vi "butterworth_lpf_tester.vi"() -> ()   [LabVIEW 2015]
uses:
  discrete_control_systems/discrete_control_systems.lvlib
  <vilib>/measure/NI_MABase.lvlib
  <vilib>/ptbypt/NI_PtbyPt.lvlib
panel:
  in  "Input Frequencies":T1(array[cluster])=[{"frequency"=10.0, "amplitude"=1.0, "phase"=0.0}, {"frequency"=100.0, "amplitude"=1.0, "phase"=0.0}, {"frequency"=250.0, "amplitude"=1.0, "phase"=0.0}]
  out "Frequency Chart":T2(graph)=[{[0.0, 1.0, 2.0, 3.0, 4.0, 5.0, 6.0, 7.0, 8.0, 9.0, 10.0, 11.0, 12.0, 13.0, 14.0, 15.0, 16.0, 17.0, 18.0, 19.0, 20.0, 21.0, 22.0, 23.0, 24.0, 25.0, 26.0, 27.0, 28.0, 29.0, 30.0, 31.0, 32.0, 33.0, 34.0, 35.0, 36.0, 37.0, 38.0, 39.0, 40.0, 41.0, 42.0, 43.0, 44.0, 45.0, 46.0, 47.0, 48.0, 49.0, 50.0, 51.0, 52.0, 53.0, 54.0, 55.0, 56.0, 57.0, 58.0, 59.0, 60.0, 61.0, 62.0, 63.0, 64.0, 65.0, 66.0, 67.0, 68.0, 69.0, 70.0, 71.0, 72.0, 73.0, 74.0, 75.0, 76.0, 77.0, 78.0, 79.0, 80.0, 81.0, 82.0, 83.0, 84.0, 85.0, 86.0, 87.0, 88.0, 89.0, 90.0, 91.0, 92.0, 93.0, 94.0, 95.0, 96.0, 97.0, 98.0, 99.0, 100.0, 101.0, 102.0, 103.0, 104.0, 105.0, 106.0, 107.0, 108.0, 109.0, 110.0, 111.0, 112.0, 113.0, 114.0, 115.0, 116.0, 117.0, 118.0, 119.0, 120.0, 121.0, 122.0, 123.0, 124.0, 125.0, 126.0, 127.0, 128.0, 129.0, 130.0, 131.0, 132.0, 133.0, 134.0, 135.0, 136.0, 137.0, 138.0, 139.0, 140.0, 141.0, 142.0, 143.0, 144.0, 145.0, 146.0, 147.0, 148.0, 149.0, 150.0, 151.0, 152.0, 153.0, 154.0, 155.0, 156.0, 157.0, 158.0, 159.0, 160.0, 161.0, 162.0, 163.0, 164.0, 165.0, 166.0, 167.0, 168.0, 169.0, 170.0, 171.0, 172.0, 173.0, 174.0, 175.0, 176.0, 177.0, 178.0, 179.0, 180.0, 181.0, 182.0, 183.0, 184.0, 185.0, 186.0, 187.0, 188.0, 189.0, 190.0, 191.0, 192.0, 193.0, 194.0, 195.0, 196.0, 197.0, 198.0, 199.0, 200.0, 201.0, 202.0, 203.0, 204.0, 205.0, 206.0, 207.0, 208.0, 209.0, 210.0, 211.0, 212.0, 213.0, 214.0, 215.0, 216.0, 217.0, 218.0, 219.0, 220.0, 221.0, 222.0, 223.0, 224.0, 225.0, 226.0, 227.0, 228.0, 229.0, 230.0, 231.0, 232.0, 233.0, 234.0, 235.0, 236.0, 237.0, 238.0, 239.0, 240.0, 241.0, 242.0, 243.0, 244.0, 245.0, 246.0, 247.0, 248.0, 249.0, 250.0, 251.0, 252.0, 253.0, 254.0, 255.0, 256.0, 257.0, 258.0, 259.0, 260.0, 261.0, 262.0, 263.0, 264.0, 265.0, 266.0, 267.0, 268.0, 269.0, 270.0, 271.0, 272.0, 273.0, 274.0, 275.0, 276.0, 277.0, 278.0, 279.0, 280.0, 281.0, 282.0, 283.0, 284.0, 285.0, 286.0, 287.0, 288.0, 289.0, 290.0, 291.0, 292.0, 293.0, 294.0, 295.0, 296.0, 297.0, 298.0, 299.0, 300.0, 301.0, 302.0, 303.0, 304.0, 305.0, 306.0, 307.0, 308.0, 309.0, 310.0, 311.0, 312.0, 313.0, 314.0, 315.0, 316.0, 317.0, 318.0, 319.0, 320.0, 321.0, 322.0, 323.0, 324.0, 325.0, 326.0, 327.0, 328.0, 329.0, 330.0, 331.0, 332.0, 333.0, 334.0, 335.0, 336.0, 337.0, 338.0, 339.0, 340.0, 341.0, 342.0, 343.0, 344.0, 345.0, 346.0, 347.0, 348.0, 349.0, 350.0, 351.0, 352.0, 353.0, 354.0, 355.0, 356.0, 357.0, 358.0, 359.0, 360.0, 361.0, 362.0, 363.0, 364.0, 365.0, 366.0, 367.0, 368.0, 369.0, 370.0, 371.0, 372.0, 373.0, 374.0, 375.0, 376.0, 377.0, 378.0, 379.0, 380.0, 381.0, 382.0, 383.0, 384.0, 385.0, 386.0, 387.0, 388.0, 389.0, 390.0, 391.0, 392.0, 393.0, 394.0, 395.0, 396.0, 397.0, 398.0, 399.0, 400.0, 401.0, 402.0, 403.0, 404.0, 405.0, 406.0, 407.0, 408.0, 409.0, 410.0, 411.0, 412.0, 413.0, 414.0, 415.0, 416.0, 417.0, 418.0, 419.0, 420.0, 421.0, 422.0, 423.0, 424.0, 425.0, 426.0, 427.0, 428.0, 429.0, 430.0, 431.0, 432.0, 433.0, 434.0, 435.0, 436.0, 437.0, 438.0, 439.0, 440.0, 441.0, 442.0, 443.0, 444.0, 445.0, 446.0, 447.0, 448.0, 449.0, 450.0, 451.0, 452.0, 453.0, 454.0, 455.0, 456.0, 457.0, 458.0, 459.0, 460.0, 461.0, 462.0, 463.0, 464.0, 465.0, 466.0, 467.0, 468.0, 469.0, 470.0, 471.0, 472.0, 473.0, 474.0, 475.0, 476.0, 477.0, 478.0, 479.0, 480.0, 481.0, 482.0, 483.0, 484.0, 485.0, 486.0, 487.0, 488.0, 489.0, 490.0, 491.0, 492.0, 493.0, 494.0, 495.0, 496.0, 497.0, 498.0, 499.0], "Power Spectrum (V^2 rms)"=[1.4416926080979755e-33, 7.826213800029281e-32, 3.9498488932288474e-32, 1.5451857789689928e-30, 1.770229960057915e-30, 1.69201989203789e-30, 2.7845850463504282e-30, 1.2307395944615857e-30, 3.884995553910035e-30, 5.168656132569903e-30, 0.4999999999999982, 1.969530656783117e-30, 1.1641495015956739e-32, 3.1610194499986036e-31, 3.906328330722268e-31, 1.457117797023426e-31, 1.330337649829857e-32, 6.461483253768492e-32, 1.5616698776899155e-32, 2.276840543231828e-32, 4.340384191049091e-32, 1.4612569748456343e-34, 2.009475244629669e-32, 1.6938033089417007e-32, 1.4069965949652836e-33, 2.9370893875103904e-34, 4.1778135170234854e-33, 5.139983465340829e-34, 3.565651291595972e-33, 1.1319414432831867e-33, 2.582687462864579e-33, 1.640047984930311e-33, 2.416435027087375e-33, 7.474025668657131e-34, 3.12677345736095e-33, 8.987590900801263e-33, 4.044144734420147e-34, 1.5808341132307828e-33, 1.5363072292167516e-32, 8.760300352472517e-34, 1.0177291753475116e-33, 5.3933988681594166e-33, 3.094430160245811e-33, 3.6514645669450685e-33, 1.845402037107353e-32, 5.966999353874168e-33, 8.386682269210854e-33, 7.536783251449749e-33, 2.7856650715616583e-33, 2.3536577227703477e-32, 6.94276482685008e-33, 7.125879164475322e-33, 4.4450660331730737e-32, 1.8424832517557833e-33, 3.2394696332391185e-32, 2.640596016281803e-32, 2.2137409152759435e-34, 2.984628117807155e-32, 3.715251366702514e-32, 8.523642080910707e-34, 3.518950726006882e-32, 3.0788156447005256e-32, 5.90445131225627e-33, 4.2742949035156564e-32, 4.4677630405293677e-32, 4.05918239542787e-33, 1.7399436600285105e-32, 3.7431449952700253e-32, 7.361354144680187e-33, 3.5112815188938977e-32, 7.714825459987569e-32, 9.56888278033162e-33, 6.891617057911108e-32, 2.901196216321453e-32, 9.942728893693235e-33, 6.820067373804319e-32, 7.66222569392888e-32, 9.778702524795351e-32, 7.459172896931001e-33, 2.6676613409008465e-32, 1.6078486549320684e-31, 4.553433334830302e-32, 5.967202732078624e-32, 1.6239147933409942e-31, 1.3496976214819333e-31, 3.9429831840891685e-32, 2.3879660230913693e-31, 5.368439062607186e-31, 5.768466483336905e-32, 1.2470806227799778e-32, 2.766251451204196e-31, 8.868922801342348e-31, 8.58630352129632e-31, 1.5210185871820127e-30, 1.3258487785965978e-30, 1.6197385144063318e-31, 1.2762558791513746e-30, 6.710012230270998e-30, 5.676225100951419e-30, 4.425084386122248e-29, 0.5000000000000158, 6.085550406083389e-29, 2.182023700085748e-29, 1.2206187767518531e-30, 2.0864465725220987e-30, 1.4770434620635963e-30, 3.523858426916773e-31, 7.93604350496358e-31, 2.565118914205842e-30, 1.7242628308667189e-31, 9.68545103065377e-31, 9.86323883154825e-32, 6.458420254775134e-31, 8.523139182093401e-32, 4.194413122625809e-31, 2.464847420841163e-31, 8.543898549846276e-32, 7.219309877932933e-32, 1.7906708675007333e-31, 4.6452074403981264e-32, 3.8477405557390846e-32, 3.035835051322331e-32, 1.2180170148794037e-31, 1.1146429562259039e-31, 6.476548031864476e-33, 8.650352863814154e-32, 4.792823037283406e-33, 7.436692826321392e-32, 1.2241937957673477e-32, 6.632121263130577e-32, 2.1380324550874632e-32, 4.143580651523067e-32, 8.799053144455967e-33, 1.0088347686413651e-32, 2.6983874731607125e-32, 6.628822838476204e-33, 2.6184364204135304e-32, 1.894787194962421e-32, 3.739693728815509e-33, 1.3373978008557082e-32, 6.624089673048897e-33, 4.0400771703784884e-33, 1.287914035386759e-33, 9.436354148245546e-33, 2.207627243261181e-33, 4.851741086145017e-34, 1.6218980211328037e-32, 6.589281185598417e-33, 1.7013683617642901e-32, 1.7443686766707493e-33, 5.763245210217634e-33, 5.65694620323976e-33, 8.631025771627826e-33, 2.5687283226277784e-33, 3.058043950990904e-33, 4.921629231963812e-33, 2.908234334710245e-33, 1.0920694549037408e-32, 3.462507728241332e-33, 1.107711087540309e-32, 5.609195466569585e-33, 6.162975822032968e-33, 6.76943729482967e-33, 6.812011131805112e-33, 5.5029211115021525e-33, 5.448070626678333e-33, 8.878235057809582e-33, 8.698966417095313e-33, 7.08882735383515e-33, 9.322166532213402e-33, 6.581787007004258e-33, 8.351078757892759e-33, 1.0268010757578787e-32, 1.1593617553095322e-32, 1.4267436939442722e-32, 6.226503776805651e-33, 9.345832359376988e-33, 1.1140811393499788e-32, 1.77715570804321e-32, 9.407881199960675e-33, 1.2642383474696908e-32, 2.2352990047032125e-32, 3.1882429782110666e-32, 4.0355165682688926e-33, 5.641464807976526e-33, 1.8364607917827892e-32, 3.5793700757787525e-32, 2.5934048778155828e-33, 1.283400271894388e-32, 3.2980721377406254e-32, 4.3911769725817854e-32, 4.6509513338604736e-33, 5.789672050545613e-33, 3.850282166966283e-32, 3.0009476777849937e-32, 9.266058800347179e-32, 3.6934714101451646e-33, 2.0164591288312445e-32, 5.897082858367753e-32, 9.435373618795044e-32, 5.983023091011311e-33, 2.8825575285456224e-32, 3.8039390539710766e-32, 1.4219318889417639e-31, 3.8445197845675e-33, 1.3808868397449647e-32, 9.7431723528794e-32, 1.2597261247197579e-31, 6.33494749937893e-33, 2.9949720564266167e-32, 7.733736551282448e-32, 1.5366164873435718e-31, 6.166451740396937e-33, 9.815204597979901e-33, 4.5732337435516326e-32, 1.6006431501198883e-31, 2.83957311411483e-31, 1.2373141549941634e-32, 7.202349368473215e-32, 2.0919361076481724e-31, 3.6135272599380592e-31, 6.013674651267553e-32, 7.876554887792541e-32, 2.1434495259467614e-31, 3.950611530668476e-31, 6.767304905202559e-32, 1.5526430748574623e-31, 2.849409038635409e-31, 5.417340072484559e-31, 3.542820085445006e-32, 1.6060656443977058e-31, 3.6131797297322066e-31, 7.814181997951294e-31, 6.70720664647277e-32, 1.1879744953070144e-31, 4.596993494460398e-31, 1.2844556938306713e-30, 2.4927911929223084e-30, 1.1357135696714613e-31, 6.407145162612521e-31, 2.1402927669151867e-30, 5.0308870470392406e-30, 2.170587773976856e-31, 1.4119777477564536e-30, 5.8193305652020806e-30, 1.7031719486667104e-29, 1.607219724884636e-30, 8.765652428972398e-30, 4.1926305807156045e-29, 3.6426071997166952e-28, 0.49999999999999956, 3.915928597894715e-29, 3.739525641719464e-29, 4.065046972439548e-29, 1.671275554714979e-30, 2.0701970633361013e-30, 4.356912241794652e-30, 6.308425787741234e-30, 8.575400552992506e-30, 3.016109187642351e-31, 1.0047009930537242e-30, 2.1368526862571695e-30, 3.281649862910867e-30, 8.007998836129683e-32, 4.7823844969883745e-31, 9.76487434778471e-31, 1.7079840097022587e-30, 1.72527962943393e-32, 1.9609726865406507e-31, 5.857500529853116e-31, 1.3969367464170784e-30, 2.2947224175787007e-33, 1.074143145500021e-31, 4.3685243386464885e-31, 7.196210120103431e-31, 1.952401774436985e-32, 7.186988767530748e-32, 1.2087302115028595e-31, 5.367618647260577e-31, 8.8410306518793e-31, 1.4671241278284904e-32, 1.0150845191636451e-31, 3.302252607498708e-31, 5.938041009600149e-31, 1.0121640081811756e-33, 5.182027286400395e-32, 1.8853293073773088e-31, 4.021625713805399e-31, 4.446241928957709e-33, 8.827188361664265e-32, 1.786214851092381e-31, 2.90188918132142e-31, 7.679961505752472e-33, 2.7273485291432385e-32, 6.905792518602725e-32, 1.4466229887560825e-31, 1.624599869735816e-32, 5.767525396924394e-32, 9.574277233070106e-32, 1.8275265106221325e-31, 2.4933813209700725e-31, 6.638289169338685e-33, 1.0338626134545707e-31, 1.4287870902078057e-31, 2.699422113541103e-31, 1.9937004917159437e-32, 2.0046237500631478e-32, 1.1164127163622637e-31, 1.3882157273333432e-31, 1.4884942464895473e-32, 5.860970285231496e-32, 9.569062739220398e-32, 1.1940654721646122e-31, 5.163513707029793e-33, 9.952195224566473e-33, 5.0014890726683e-32, 9.387792363967579e-32, 5.844103453009723e-33, 2.529090527327928e-32, 6.281038717263985e-32, 7.85497399535959e-32, 2.2036920599380478e-31, 2.4715998236716116e-31, 3.649055829476238e-31, 5.747485248453361e-32, 1.5857090271070457e-32, 2.159038341881439e-33, 7.128171791486171e-33, 3.5622000251406624e-32, 8.174423218938077e-32, 2.080194652630683e-31, 3.1555668804010515e-31, 2.5174622245462084e-32, 2.8246150787582163e-32, 2.527904770782537e-33, 8.297732039181169e-33, 5.646557891196919e-32, 3.399115358937183e-32, 1.430387491767795e-31, 2.2816827933350695e-31, 8.26204840916961e-32, 5.89015320835258e-33, 9.591192752807049e-33, 5.116946261717839e-33, 1.7254360149465082e-32, 8.958817199272511e-32, 9.71892412450502e-32, 7.57218954755664e-32, 2.5206977868567314e-31, 6.142763726532455e-32, 1.866634721406879e-32, 3.5498740734961555e-36, 3.415671577183976e-32, 2.8554102363468444e-32, 5.553827291790369e-32, 5.395663145483737e-32, 1.3876743715382034e-31, 5.687785734253585e-32, 2.6963758778492407e-32, 4.258493033511518e-33, 3.909791861504521e-33, 1.0033447897801486e-32, 8.036993788484802e-32, 7.705122470851042e-32, 1.679706734345367e-31, 1.451790027684439e-31, 7.869208004324589e-33, 6.816867556754343e-33, 3.537646729466782e-33, 2.628168991832792e-32, 4.0174837010141386e-32, 5.169957714550326e-32, 1.527650097078272e-31, 1.3031518698467966e-31, 3.2384145317808095e-32, 6.312169140739151e-33, 5.3999747633671905e-33, 2.189296087975849e-32, 1.4354113031403455e-32, 3.514947256913391e-32, 1.089450683217444e-31, 1.244847160341577e-31, 2.6802042292968876e-32, 2.5341490978820214e-32, 2.0180048031687845e-33, 1.7946807460909326e-32, 1.1743180650352467e-32, 2.2427044364487333e-32, 5.072424924381758e-32, 8.90328139154572e-32, 9.703159232348172e-32, 2.1588066139879466e-32, 1.7463211074103228e-32, 1.0626942469462871e-33, 5.999607658948919e-33, 3.8838975022852487e-32, 4.0559776479980306e-32, 5.512582192397203e-32, 9.454073936344552e-32, 1.2164629588961027e-32, 1.7798797433566294e-32, 7.2774883697011045e-34, 1.1938670243423738e-33, 2.8224777587405567e-32, 2.204779948430053e-32, 5.080579773987662e-32, 7.21580930767338e-32, 1.5983961291342411e-31, 2.205420897918006e-32, 3.9304994602634846e-33, 3.3588218230124426e-34, 2.4496349778408686e-33, 2.968661080051771e-32, 5.078511479299452e-32, 4.219902944103315e-32, 8.313114826831756e-32, 7.485229958705841e-33, 2.9408734546643856e-33, 1.7258797492053588e-34, 9.788901017172564e-33, 1.4031666136383775e-32, 2.7729077116113653e-32, 5.037872816731285e-32, 8.148311922976104e-32, 1.4448480517192225e-32, 1.2947672644997138e-32, 1.144045527797009e-33, 3.486765201078367e-34, 3.9629413649927634e-33, 2.8357380175181866e-32, 4.0552306953291036e-32, 4.6022367077709563e-32, 7.191699746252629e-32, 1.292975071131367e-32, 7.59456114979016e-33, 1.874752593161026e-33, 7.849659045018005e-33, 1.0383381664975952e-32, 2.571501661748799e-32, 3.739299298360432e-32, 5.668951680141826e-32, 8.255922411207759e-33, 9.679816345129692e-33, 1.0653566524999264e-32, 3.642885704599775e-33, 1.2703939277186302e-32, 3.024029254835997e-32, 4.8065294955136534e-32, 6.813966027738547e-32, 8.356936666421175e-32, 1.2133469583202118e-32, 1.3503844235078742e-32, 2.512084411845396e-33, 9.571403437448685e-33, 1.1312758418942347e-32, 2.825909303677101e-32, 4.027135537450095e-32, 9.253112237036031e-32, 1.0464461774891864e-32, 1.5176327961762745e-32, 7.089418999507104e-33, 8.293202251943456e-33, 1.1924150272388417e-32, 2.195261848573145e-32, 4.047611408325447e-32, 6.380061098690229e-32, 1.8233163969520864e-32, 1.0734480234574379e-32, 2.7900284584438765e-33, 2.1033065515213554e-33, 7.669509098764695e-33, 1.3050224562689651e-32, 3.675588919504871e-32, 5.450871699191517e-32, 7.812854369708136e-32, 2.058380306669531e-32, 1.1337153017972642e-32, 7.552149090920312e-33, 7.651742780204426e-33, 1.379131624231117e-32, 2.636753400858088e-32, 4.5377867718164147e-32, 6.998247016682413e-32, 1.5021552527732508e-32, 6.02551680930733e-33, 4.0678490801767065e-33, 1.073269913457202e-33, 1.0601281378875458e-32, 1.884817695643121e-32, 3.6690863637132524e-32, 4.0766899075114406e-32, 8.618009566694101e-32, 1.2294406837513389e-32, 4.4976180361500075e-33, 6.401820505569718e-33, 3.665055565675666e-33, 1.8815563740220795e-32, 3.133180034428294e-32, 4.5617842079968393e-32, 6.914593886032232e-32]}, ...(2 in all)]
  out "Time Chart":cluster{dbl, "y(k)":dbl}(graph)={-0.8257232827308646, "y(k)"=-0.15972354896016128}
  in  "Reset? (F)":bool
  in  "Sampling Time (s)":dbl=0.001
  in  "Cut Off Frequency (Fc in Hz)":dbl=150.0
  in  "Stop":bool
  # "JKI DISCRETE CONTROL SYSTEMS\nLow Pass Filter Example\nThis example shows how to use the low pass filter (LPF) in order to remove noise from an input signal. A LPF \ncould be useful inline as part of a control loop to remove sensor noise"
  # "Filter Configuration"
  # "Set Before Running"
  # "Set the cutoff frequency of the low pass filter.\nThis is settable while running without resetting"
  # "Select the frequencies for the input signal"
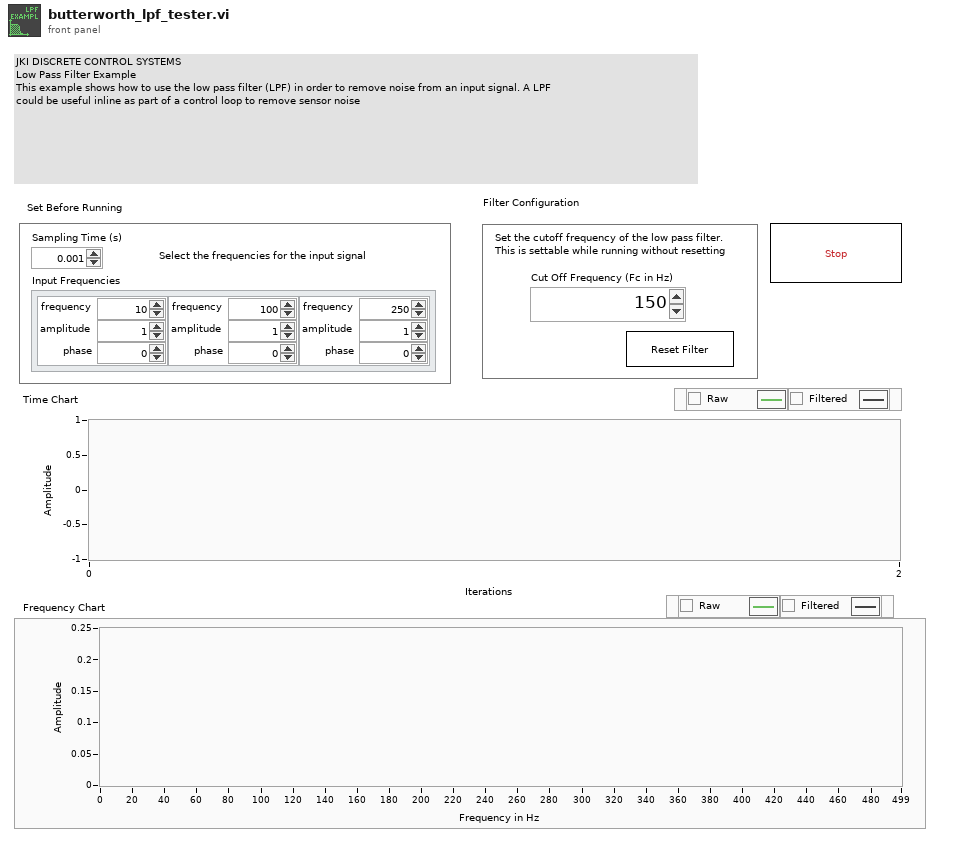
[diagram p1: front panel]
types:
  T1 = cluster{"frequency":dbl, "amplitude":dbl, "phase":dbl}[]
  T2 = cluster{dbl[], "Power Spectrum (V^2 rms)":dbl[]}[]
  T3 = enum8{"Enabled", "Disabled", "Disabled and Grayed Out"}
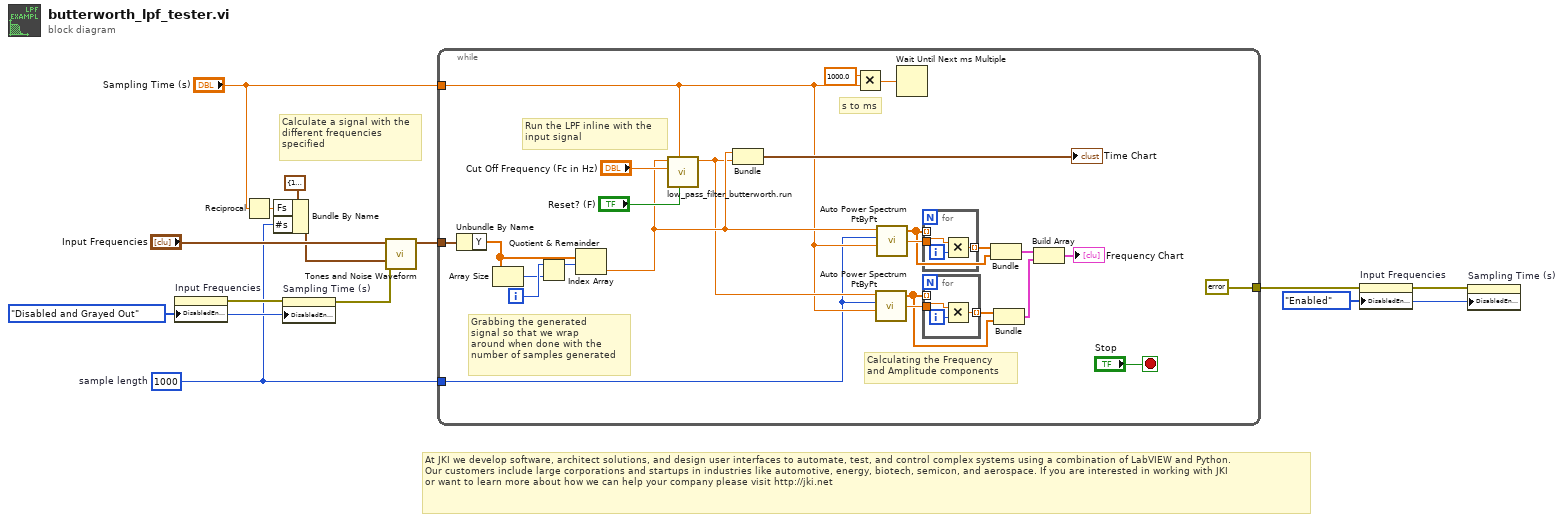
[diagram p0: block diagram]
diagram:
  w1 = 1000  # sample length
  w4 = T3."Enabled" ("Disabled")
  w5 = T3."Disabled and Grayed Out" ("Disabled")
  # "At JKI we develop software, architect solutions, and design user interfaces to automate, test, and control complex systems using a combination of LabVIEW and Python. \nOur customers include large corporations and startups in industries like automotive, energy, biotech, semicon, and aerospace. If you are interested in working with JKI\nor want to learn more about how we can help your company please visit http://jki.net"
  # "Calculate a signal with the\ndifferent frequencies\nspecified"
  n1 = property on="Input Frequencies" class="Arr (strict)"("DisabledEnum"=w5) -> (error out=w7:errorcluster)  [unwired: 2 in, 1 out]
  n2 = Reciprocal(x="Sampling Time (s)") -> (1/x=w8:dbl)
  n3 = Bundle By Name(cluster=cluster{"Fs":dbl, "#s":dbl} {"Fs"=100.0, "#s"=1000.0} ("sampling info"), "Fs"=w8, "#s"=w1) -> (w10:cluster{"Fs":dbl, "#s":dbl})
  n4 = property on="Sampling Time (s)" class="DigNum (strict)"(error in=w7, "DisabledEnum"=w5) -> (error out=w6:errorcluster)  [unwired: 1 in, 1 out]
  n5 = call <vilib>:"Tones and Noise Waveform.vi"("sampling info"=w10, "error in (no error)"=w6, "tones"="Input Frequencies") -> ("signal out"=w12:waveform(dbl))  [unwired: 7 in, 1 out]
  n6 = while {
    tunnel: w12 -> [w33]
    tunnel: "Sampling Time (s)" -> [w16]
    tunnel: [errorcluster {"status"=FALSE, "code"=0, "source"=""} ("error in (no error)")] -> w2
    tunnel: w1 -> [w14]
    i -> [w30]
    stop <- "Stop" stop-if-true
    # "Run the LPF inline with the\ninput signal"
    # "Grabbing the generated\nsignal so that we wrap\naround when done with the\nnumber of samples generated"
    # "Calculating the Frequency\nand Amplitude components"
    # "s to ms"
    n7 = Unbundle By Name(w33) -> ("Y"=w32:dbl[])
    n8 = Array Size(array=w32) -> (size(s)=w29:i32)
    n9 = Quotient & Remainder(x=w30, y=w29) -> (x-y*floor(x/y)=w28:i32)  [unwired: 1 out]
    n10 = Index Array(array=w32, index=w28) -> (element=w27:dbl)
    n11 = call "low_pass_filter_butterworth.run.vi"("Reset? (F)"="Reset? (F)", "sampling_time (s)"=w16, "cuttoff_frequency (fc in Hz)"="Cut Off Frequency (Fc in Hz)", "input"=w27) -> ("output"=w26:dbl)  [unwired: 7 in]
    n12 = Bundle(w27, "output"=w26) -> (→"Time Chart":cluster{dbl, "output":dbl})  [unwired: 1 in]
    n13 = Multiply(x=1000.0, y=w16) -> (x*y=w34:dbl)
    n14 = call <vilib>:"Auto Power Spectrum PtByPt.vi"("signal"=w26, "sample length"=w14, "dt"=w16) -> ("Power Spectrum (V^2 rms)"=w19:dbl[], "df"=w21:dbl)  [unwired: 2 in, 1 out]
    n15 = call <vilib>:"Auto Power Spectrum PtByPt.vi"("signal"=w27, "sample length"=w14, "dt"=w16) -> ("Power Spectrum (V^2 rms)"=w23:dbl[], "df"=w25:dbl)  [unwired: 2 in, 1 out]
    n16 = Wait Until Next ms Multiple(millisecond multiple=w34) -> ()  [unwired: 1 out]
    n17 = for {
      tunnel: w25 -> [w41]
      tunnel: w23 -> [_] mode=indexing
      tunnel: [w39] -> w24 mode=indexing
      i -> [w40]
      n18 = Multiply(x=w41, y=w40) -> (x*y=w39:dbl)
    }
    n19 = for {
      tunnel: w21 -> [w44]
      tunnel: [w42] -> w20 mode=indexing
      tunnel: w19 -> [_] mode=indexing
      i -> [w43]
      n20 = Multiply(x=w44, y=w43) -> (x*y=w42:dbl)
    }
    n21 = Bundle(w24, "Power Spectrum (V^2 rms)"=w23) -> (w22:cluster{dbl[], "Power Spectrum (V^2 rms)":dbl[]})  [unwired: 1 in]
    n22 = Bundle(w20, "Power Spectrum (V^2 rms)"=w19) -> (w18:cluster{dbl[], "Power Spectrum (V^2 rms)":dbl[]})  [unwired: 1 in]
    n23 = Build Array(w22, w18) -> (→"Frequency Chart":T2)
  }
  n24 = property on="Input Frequencies" class="Arr (strict)"(error in=w2, "DisabledEnum"=w4) -> (error out=w3:errorcluster)  [unwired: 1 in, 1 out]
  n25 = property on="Sampling Time (s)" class="DigNum (strict)"(error in=w3, "DisabledEnum"=w4) -> ()  [unwired: 1 in, 2 out]
